vi "oa_IIR Param Change Check.vi"(0 "design method in":u16, 1 "filter type in":T1(ring), 5 "sampling freq in":dbl, 7 "freq specs in":cluster{"low cutoff":dbl, "high cutoff":dbl}={"low cutoff"=0.12500000000000006, "high cutoff"=0.45000000000000007} {"high cutoff" format="%0.2f"; "low cutoff" format="%0.4f"}, 9 "ripple specs in [dB]":cluster{"pass band":dbl, "stop band":dbl}={"pass band"=0.1, "stop band"=60.0} {"stop band" format="%0.2f"; "pass band" format="%0.2f"}, 11 "order in":i32) -> (3 "filter type out":T1(ring), 4 "design method out":u16, 6 "sampling freq out":dbl, 8 "freq specs out":cluster{"low cutoff":dbl, "high cutoff":dbl}, 10 "ripple specs out [dB]":cluster{"pass band":dbl, "stop band":dbl}, 14 "chang?":bool, 15 "order out":i32)   [LabVIEW 2017, in "SoundVib_RefDataProcess.lvlib"]
uses:
  <vilib>/addons/Sound and Vibration/Order Analysis/Referece Data Processing/SoundVib_RefDataProcess.lvlib
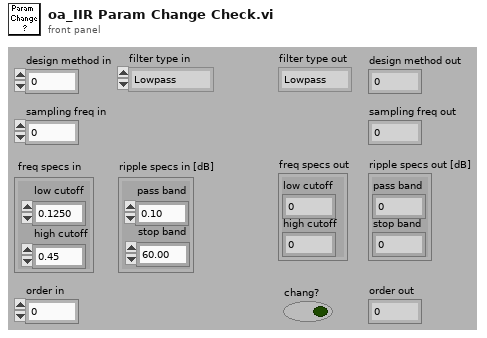
[diagram p1: front panel]
types:
  T1 = enum32{"Lowpass", "Highpass", "Bandpass", "Bandstop"}
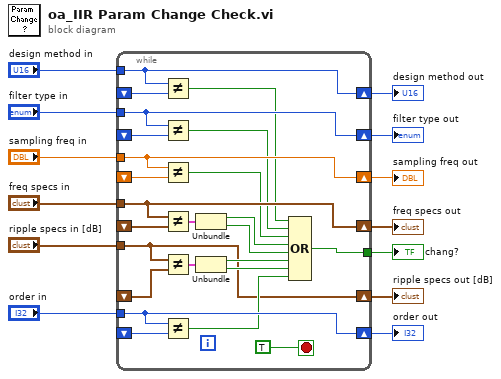
[diagram p0: block diagram]
diagram:
  n1 = while {
    shift-right: [w34] -> w9
    shift-left: _ -> [w33]
    shift-right: [w32] -> w2
    shift-left: _ -> [w31]
    shift-right: [w14] -> w1
    shift-left: _ -> [w30]
    shift-right: [w28] -> w8
    shift-left: _ -> [w29]
    shift-right: [w36] -> w13
    shift-left: _ -> [w35]
    tunnel: "design method in" -> [w36]
    tunnel: "filter type in" -> [w34]
    tunnel: "freq specs in" -> [w32]
    tunnel: "ripple specs in [dB]" -> [w14]
    tunnel: "order in" -> [w28]
    tunnel: [w27] -> w3
    tunnel: "sampling freq in" -> [w25]
    shift-right: [w25] -> w6
    shift-left: _ -> [w26]
    stop <- TRUE stop-if-true
    n2 = Not Equal?(x=w36, y=w35) -> (x != y?=w24:bool)
    n3 = Not Equal?(x=w34, y=w33) -> (x != y?=w23:bool)
    n4 = Not Equal?(x=w25, y=w26) -> (x != y?=w22:bool)
    n5 = Not Equal?(x=w32, y=w31) -> (x != y?=w21:cluster{"low cutoff":bool, "high cutoff":bool})
    n6 = Not Equal?(x=w14, y=w30) -> (x != y?=w20:cluster{"pass band":bool, "stop band":bool})
    n7 = Not Equal?(x=w28, y=w29) -> (x != y?=w15:bool)
    n8 = Unbundle(w21) -> ("low cutoff"=w19:bool, "high cutoff"=w18:bool)
    n9 = Unbundle(w20) -> ("pass band"=w17:bool, "stop band"=w16:bool)
    n10 = Compound Arithmetic op=OR(w24, w23, w22, w19, w18, w17, w16, w15) -> (w27:bool)
  }
  "design method out" <- w13
  "chang?" <- w3
  "filter type out" <- w9
  "order out" <- w8
  "sampling freq out" <- w6
  "freq specs out" <- w2
  "ripple specs out [dB]" <- w1
